vi "splash_demo_v1.0.vi"() -> ()   [LabVIEW 2025]
doc: "Proof of concept/example VI for demonstration.\n\nMichael Panganiban\nSr. Hardware Test Engineer\nFresh Consulting, Inc."
uses:
  controls/home_navigation_btn.ctl
  controls/equipment_navigation_btn.ctl
  controls/settings_navigation_btn.ctl
  controls/test_plan_navigation_btn.ctl
  controls/queue_data.ctl
panel:
  in  "test_plan":T1
  in  "settings":T2
  in  "equipment":T3
  in  "home":T4
  in  "Tab":T5(tab)
  # "v1.0.0.1"
  # "HOME"
  # "EQUIPMENT"
  # "SETTINGS"
  # "TEST PLAN CREATION"
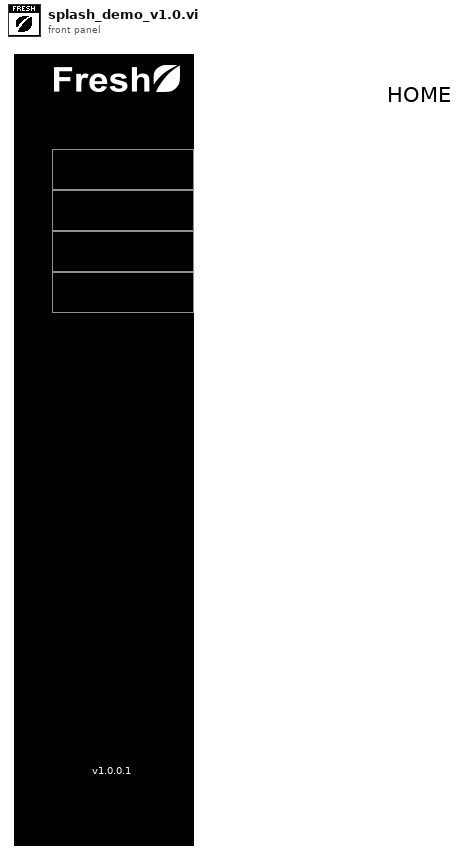
[diagram p1: front panel]
types:
  T1 = typedef "test_plan_navigation_btn.ctl" = bool
  T2 = typedef "settings_navigation_btn.ctl" = bool
  T3 = typedef "equipment_navigation_btn.ctl" = bool
  T4 = typedef "home_navigation_btn.ctl" = bool
  T5 = enum32{"home", "equipment", "settings", "test_plan"}
  T6 = typedef "queue_data.ctl" = cluster{"Action":string, "btn_ref":refnum<vi>}
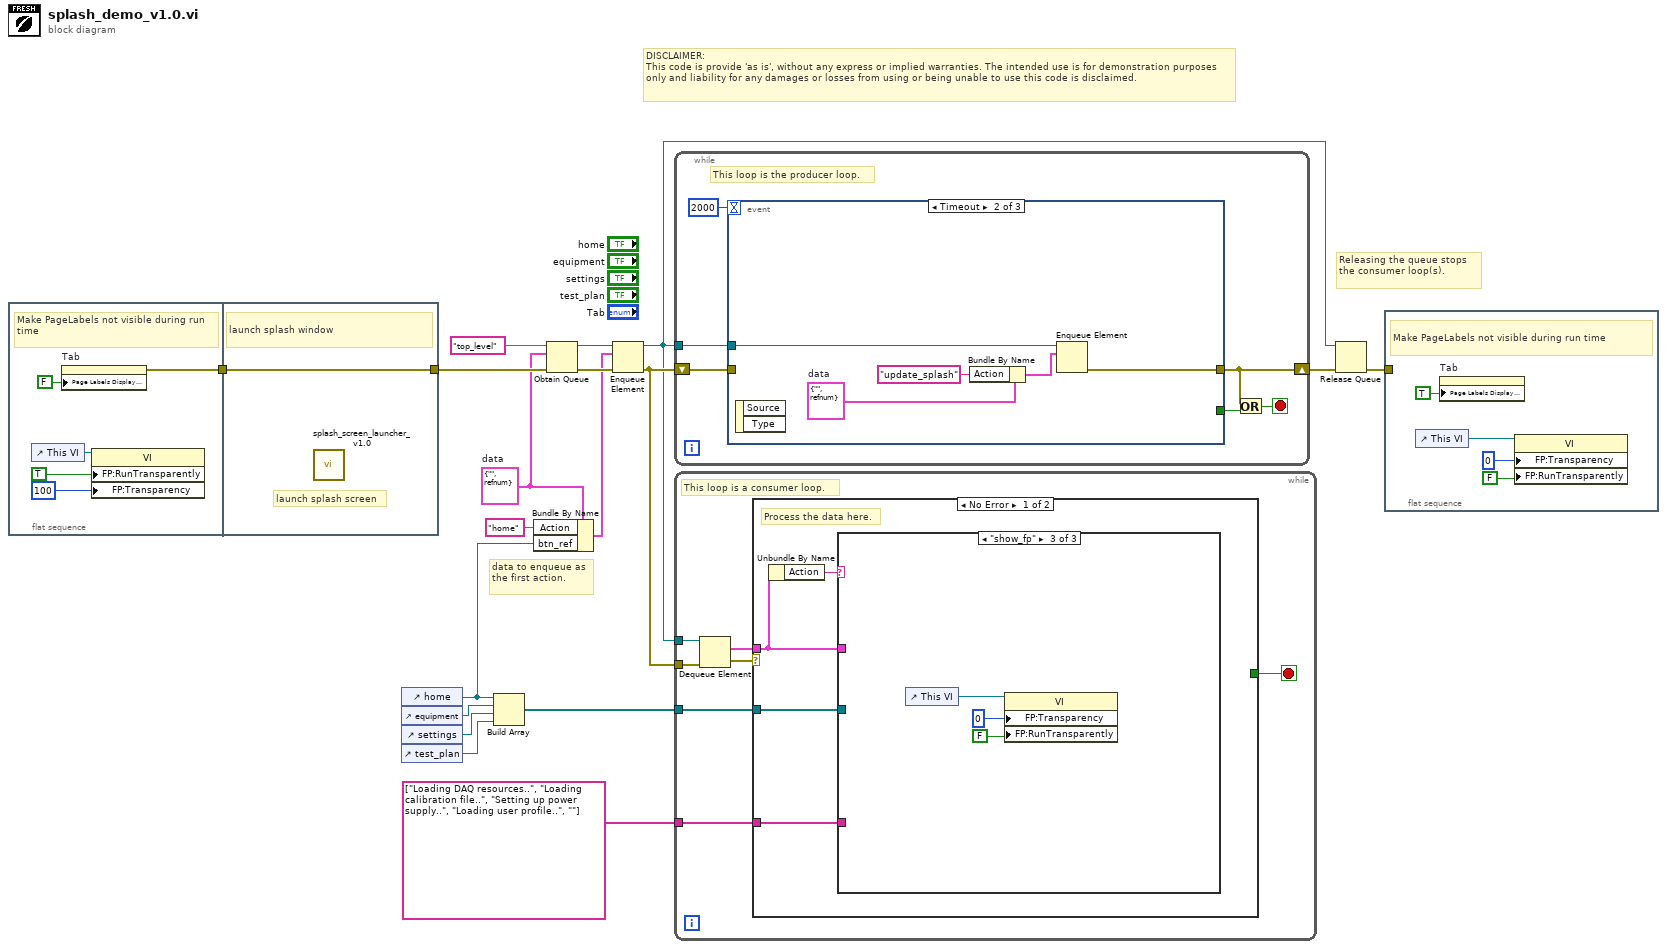
[diagram p0: block diagram]
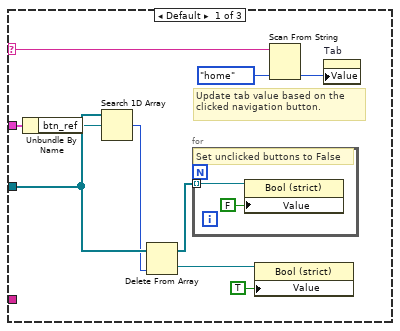
[diagram p2: hidden frame]
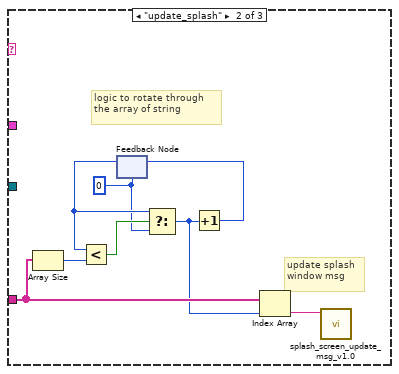
[diagram p3: hidden frame]
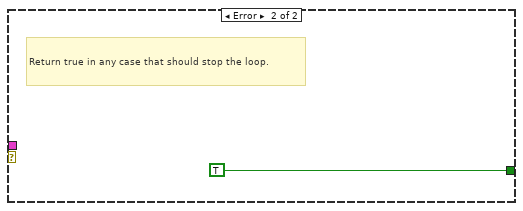
[diagram p4: hidden frame]
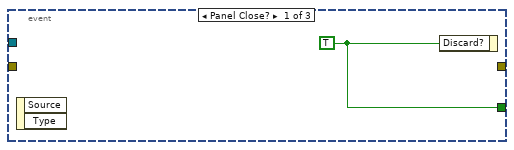
[diagram p5: hidden frame]
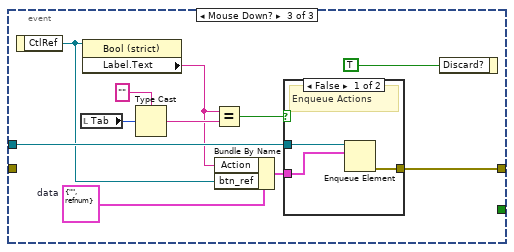
[diagram p6: hidden frame]
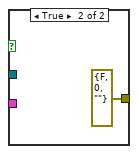
[diagram p7: hidden frame]
diagram:
  w9 = T6 {"Action"="", "btn_ref"=refnum}  # data
  # "data to enqueue as the first action."
  # "DISCLAIMER:\nThis code is provide 'as is', without any express or implied warranties. The intended use is for demonstration purposes only and liability for any damages or losses from using or being unable to use this code is disclaimed."
  # "Releasing the queue stops the consumer loop(s)."
  n1 = flat-sequence {
    tunnel: [w22] -> w2
    tunnel: [w24] -> w17
    tunnel: w2 -> [w24]
    frame #0 {
      # "Make PageLabels not visible during run time"
      n2 = control-ref of="This VI"() -> (w19:refnum<vi>)
      n3 = property on="Tab" class="TabCtl (strict)"("Page Labels Display Visible?"=FALSE) -> (error out=w22:errorcluster)  [unwired: 2 in, 1 out]
      n4 = property class="VI"(reference=w19, "FP:RunTransparently"=TRUE ("Front Panel Window:Run VI Transparently"), "FP:Transparency"=u8 100 ("Front Panel Window:Transparency")) -> ()  [unwired: 1 in, 2 out]
    }
    frame #1 {
      # "launch splash screen"
      # "launch splash window"
      n5 = call "splash_screen_launcher_v1.0.vi"() -> ()  [unwired: 11 in, 1 out]
    }
  }
  n6 = control-ref of="home"() -> (w8:refnum<vi>)
  n7 = control-ref of="equipment"() -> (w15:refnum<vi>)
  n8 = control-ref of="settings"() -> (w14:refnum<vi>)
  n9 = control-ref of="test_plan"() -> (w13:refnum<vi>)
  n10 = Build Array(w8, w15, w14, w13) -> (w12:refnum<vi>[])
  n11 = Bundle By Name(cluster=w9, "Action"="home", "btn_ref"=w8) -> (w6:T6)
  n12 = Obtain Queue(name (unnamed)="top_level", element data type=w9, error in (no error)=w17) -> (queue out=w11:refnum<queue>, error out=w10:errorcluster)  [unwired: 2 in, 1 out]
  n13 = Enqueue Element(queue=w11, element=w6, error in (no error)=w10) -> (queue out=w4:refnum<queue>, error out=w5:errorcluster)  [unwired: 1 in, 1 out]
  n14 = while {
    shift-right: [w27] -> w18
    shift-left: w5 -> [w30]
    tunnel: w4 -> [w26]
    stop <- w28 stop-if-true
    # "This loop is the producer loop."
    n15 = event shown="[1] Timeout" {
      selector: _ -> [_ _ _]
      dyn-events: _ -> [_ _ _]
      timeout: 2000 -> [_ _ _]
      tunnel: w26 -> [_ w36 w44]
      tunnel: w30 -> [_ _ _]
      tunnel: [_ w35 w45] -> w27
      tunnel: [w31 _ _] -> w29
      event Panel Close? {
        w31 = TRUE ("Discard?")
        n16 = event-data() -> ()  [unwired: 1 in, 2 out]
        n17 = event-data("Discard?"=w31) -> ()  [unwired: 1 in, 1 out]
      }
      event Timeout {
        w34 = T6 {"Action"="", "btn_ref"=refnum}  # data
        n18 = event-data() -> ()  [unwired: 1 in, 2 out]
        n19 = Bundle By Name(cluster=w34, "Action"="update_splash") -> (w33:T6)
        n20 = Enqueue Element(queue=w36, element=w33) -> (error out=w35:errorcluster)  [unwired: 2 in, 2 out]
      }
      event Mouse Down? {
        w46 = T6 {"Action"="", "btn_ref"=refnum}  # data
        n21 = event-data() -> ("CtlRef"=w43:refnum<vi>)  [unwired: 1 in]
        n22 = local read "Tab"() -> (w41:T5)
        n23 = property class="Bool (strict)"(reference=w43) -> ("Label.Text"=w38:string)  [unwired: 1 in, 2 out]
        n24 = Type Cast(type="", x=w41) -> (*(type *) &x=w39:string)
        n25 = Equal?(x=w38, y=w39) -> (x = y?=w37:bool)
        n26 = Bundle By Name(cluster=w46, "Action"=w38, "btn_ref"=w43) -> (w47:T6)
        n27 = case shown="False" w37 {
          tunnel: [w50 errorcluster {"status"=FALSE, "code"=0, "source"=""} ("error out")] -> w45
          tunnel: w44 -> [w49 _]
          tunnel: w47 -> [w48 _]
          frame False {
            # "Enqueue Actions"
            n28 = Enqueue Element(queue=w49, element=w48) -> (error out=w50:errorcluster)  [unwired: 2 in, 2 out]
          }
          frame True {
          }
        }
        n29 = event-data("Discard?"=TRUE) -> ()  [unwired: 1 in, 1 out]
      }
    }
    n30 = Or(x=w27, y=w29) -> (x .or. y?=w28:bool)
  }
  n31 = while {
    tunnel: w4 -> [w58]
    tunnel: w12 -> [w54]
    tunnel: w5 -> [w53]
    tunnel: string[] ["Loading DAQ resources..", "Loading calibration file..", "Setting up power supply..", "Loading user profile..", ""] -> [w52]
    stop <- w55 stop-if-true
    # "This loop is a consumer loop."
    n32 = Dequeue Element(queue=w58, error in (no error)=w53) -> (element=w56:T6, error out=w57:errorcluster)  [unwired: 1 in, 2 out]
    n33 = case shown="No Error" w57 {
      tunnel: w56 -> [w61 _]
      tunnel: [_ TRUE] -> w55
      tunnel: w54 -> [w62 _]
      tunnel: w52 -> [w59 _]
      frame No Error {
        # "Process the data here."
        n34 = Unbundle By Name(w61) -> ("Action"=w60:string)
        n35 = case shown="\"show_fp\"" w60 {
          selector: w60 -> [w63 _ _]
          tunnel: w61 -> [w72 _ _]
          tunnel: w62 -> [w71 _ _]
          tunnel: w59 -> [_ w80 _]
          frame Default {
            # "Update tab value based on the clicked navigation button."
            n36 = Unbundle By Name(w72) -> ("btn_ref"=w66:refnum<vi>)
            n37 = Search 1D Array(1D array=w71, element=w66) -> (index of element=w70:i32)  [unwired: 1 in]
            n38 = Delete From Array "Delete From Array"(array=w71, index=w70) -> (deleted portion=w69:refnum<vi>, array with subset deleted=w67:refnum<vi>[])  [unwired: 1 in]
            n39 = for {
              tunnel: w67 -> [w73] mode=indexing
              # "Set unclicked buttons to False"
              n40 = property class="Bool (strict)"(reference=w73, "Value"=T4 FALSE) -> ()  [unwired: 1 in, 2 out]
            }
            n41 = property class="Bool (strict)"(reference=w69, "Value"=T4 TRUE) -> ()  [unwired: 1 in, 2 out]
            n42 = Scan From String(input string=w63, default 1=T5."home" ("Tab Control")) -> (output 1=w64:T5)  [unwired: 3 in, 3 out]
            n43 = property on="Tab" class="TabCtl (strict)"("Value"=w64) -> ()  [unwired: 2 in, 2 out]
          }
          frame "update_splash" {
            w75 = 0
            # "update splash window msg"
            # "logic to rotate through the array of string"
            n44 = Array Size(array=w80) -> (size(s)=w81:i32)
            n45 = feedback #1(w75) -> (w76:i32)
            n46 = Less?(x=w76, y=w81) -> (x < y?=w82:bool)
            n47 = Select(t=w76, s=w82, f=w75) -> (s? t:f=w77:i32)
            n48 = Increment(x=w77) -> (x+1=w78:i32)
            n49 = feedback-in #1(w78) -> ()
            n50 = Index Array(array=w80, index=w77) -> (element=w79:string)
            n51 = call "splash_screen_update_msg_v1.0.vi"("message in"=w79) -> ()  [unwired: 10 in, 1 out]
          }
          frame "show_fp" {
            n52 = control-ref of="This VI"() -> (w83:refnum<vi>)
            n53 = property class="VI"(reference=w83, "FP:Transparency"=u8 0 ("Front Panel Window:Transparency"), "FP:RunTransparently"=FALSE ("Front Panel Window:Run VI Transparently")) -> ()  [unwired: 1 in, 2 out]
          }
        }
      }
      frame Error {
        # "Return true in any case that should stop the loop."
      }
    }
  }
  n54 = Release Queue(queue=w4, error in (no error)=w18) -> (error out=w16:errorcluster)  [unwired: 1 in, 2 out]
  n55 = flat-sequence {
    tunnel: w16 -> [_]
    frame #0 {
      # "Make PageLabels not visible during run time"
      n56 = control-ref of="This VI"() -> (w89:refnum<vi>)
      n57 = property on="Tab" class="TabCtl (strict)"("Page Labels Display Visible?"=TRUE) -> ()  [unwired: 2 in, 2 out]
      n58 = property class="VI"(reference=w89, "FP:Transparency"=u8 0 ("Front Panel Window:Transparency"), "FP:RunTransparently"=FALSE ("Front Panel Window:Run VI Transparently")) -> ()  [unwired: 1 in, 2 out]
    }
  }
